vi "Revision Query.vi"(8 "error in (no error)":errorcluster {"code" format="%.0x"}, 11 "instrument handle":refnum<k15>) -> (0 "error out":errorcluster {"code" format="%.0x"}, 1 "firmware revision":string, 2 "instrument driver revision":string, 3 "instrument handle out":refnum<k15>)   [LabVIEW 2021, in "Keysight XSAnVMA.lvlib"]
doc: "Retrieves revision information from the instrument."
uses:
  <instrlib>/Keysight XSAnVMA/Keysight XSAnVMA.lvlib
  KtXSAnVMA_64.dll
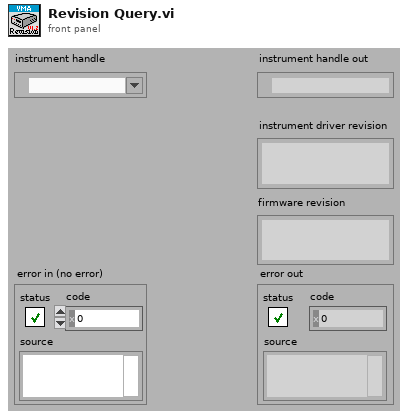
[diagram p1: front panel]
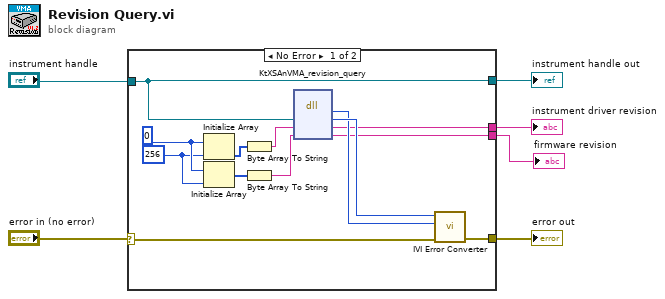
[diagram p0: block diagram]
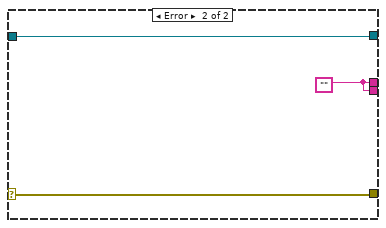
[diagram p2: hidden frame]
diagram:
  n1 = case shown="No Error" "error in (no error)" {
    selector: "error in (no error)" -> [w9 w21]
    tunnel: [w14 w21] -> w6
    tunnel: "instrument handle" -> [w10 w22]
    tunnel: [w10 w22] -> w4
    tunnel: [w8 w20] -> w2
    tunnel: [w7 w20] -> w1
    frame No Error {
      w11 = 256
      w12 = u8 0
      n2 = Initialize Array(w12, w11) -> (w19:u8[])
      n3 = Initialize Array(w12, w11) -> (w18:u8[])
      n4 = Byte Array To String(unsigned byte array=w19) -> (string=w17:string)
      n5 = Byte Array To String(unsigned byte array=w18) -> (string=w16:string)
      n6 = dll-call lib="KtXSAnVMA**.dll" fn="KtXSAnVMA_revision_query" ("LabVIEW:IviDmm_revision_query")("instrument handle"=w10, "instrument driver revision"=w17, "firmware revision"=w16) -> ("Status"=w13:i32, "instrument handle"=w15:u32, "instrument driver revision"=w8:string, "firmware revision"=w7:string)  [unwired: 3 in, 2 out]
      n7 = call <instrlib>:"IVI Error Converter.vi"("error in (no error)"=w9, "IVI error code (0)"=w13, "instrument handle"=w15) -> ("error out"=w14:errorcluster)  [unwired: 7 in, 1 out]
    }
    frame Error {
      w20 = ""
    }
  }
  "error out" <- w6
  "instrument handle out" <- w4
  "instrument driver revision" <- w2
  "firmware revision" <- w1
